vi "Test Tool Module API.vi"() -> ()   [LabVIEW 2015]
doc: "Tool Module API Tester.\n\n<b>Note:</b> This VI was modified by the <b>Validate DQMH Module</b> tool to upgrade it to the DQMH 3.0 approach to error handling in the tester VI, which avoids the potential for an error that stops the loop preventing the Stop Module VI from executing.\n\n<b>Note:</b> This VI was modified by the <b>Validate DQMH Module</b> tool to upgrade it to the DQMH 5.0 approach to only call the Stop Module.vi at the end of the tester if the module wasn't originally running when the tester started."
uses:
  Support/_STATUS Typedef--cluster.ctl
  GOTO Argument--cluster.ctl
  Support/_GoTo Cmd Typedef--enum.ctl
  Get All Inspect Data (Reply Payload)--cluster.ctl
  Tool Typedefs/_Temperature Threshold Arrays--typedef.ctl
  Return FPGA Setup Data (Reply Payload)--cluster.ctl
  Tool Typedefs/_FPGA Setup Params Cluster--typedef.ctl
  Tool Typedefs/_FPGA Timing Constraints Cluster--typedef.ctl
  Tool Typedefs/_FPGA Timing Ctrl Cluster--typedef.ctl
  Tool Typedefs/_FPGA Laser Config Cluster--typedef.ctl
  Tool Typedefs/_FPGA Peak Proc Cfg Cluster--typedef.ctl
  Tool Typedefs/_FPGA SPI Cfg Cluster--typedef.ctl
  Read from File Rtn Argument--cluster.ctl
  Tool Module.lvlib
  QC-X App/File Manager/File Manager.lvlib
panel:
  in  "Read Tool File":bool
  in  "Count":i32
  in  "Period":i32
  in  "Timer On":bool
  in  "Setup Timer 1":bool
  out "Return FPGA Setup Data":T1={"Version String"="", "FPGA Setup Parameters"={"FPGA Timing Constraints"={"frame.length Min"=530, "frame.ST_OFF Min"=15, "frame.ST_ON Min"=8, "frame.first data idx"=14, "frame.integ Offset"=6, "frame.integ Delay"=3, "frame.ad_latch Delay"=11, "frame.trig time Max"=0}, "FPGA Timing Ctrl"={"trig.time"=220, "integ.count 1"=400, "integ.count 2"=350, "encdr.latch ctrl"=1, "pixel.read count"=512, "clock.select"=2, "ad.clock offset"=16, "data.control reg"=2}, "FPGA Laser Config"={"laser.gain"=10, "laser.threshold Low"=1400, "laser.threshold High"=1900, "laser.dac init"=912, "laser.dac Min"=800, "laser.dac Max"=4000, "laser.config reg"=3}, "FPGA Peak Proc Cfg"={"PD.threshold"=0, "PD.width detect Min"=0, "PD.sensor pixels"=512, "PD.config reg"=23}, "FPGA SPI Cfg"={"SPI Divide Value"=1, "SPI config reg"=1}}, "Return FPGA Setup Data_error"={"status"=FALSE, "code"=0, "source"=""}} {"FPGA Setup Parameters"."FPGA SPI Cfg"."SPI config reg" format="%03b"; "FPGA Setup Parameters"."FPGA Peak Proc Cfg"."PD.config reg" format="%05b"; "FPGA Setup Parameters"."FPGA Laser Config"."laser.config reg" format="%02b"; "FPGA Setup Parameters"."FPGA Timing Ctrl"."data.control reg" format="%03b"; "FPGA Setup Parameters"."FPGA Timing Constraints"."frame.trig time Max" format="%0.0f"}
  in  "Return FPGA Setup Data":bool
  in  "Get Cycle Count":bool
  in  "Set Device Temp Tholds":bool
  in  "Device Temp Thold Arrays":T8
  in  "Read from File":bool
  in  "Write to File":bool
  out "error in (no error)":errorcluster
  out "XML String":string[](array[string])
  out "Waveform Graph":u16[][](graph)
  out "All Stop":bool
  out "Scan Data Array":u32[](array[numeric])
  out "Inspecting":bool
  out "Status 2":u8 format="%x"
  out "Reply Payload":T9
  out "Tool SN":u16
  out "Tool Type":u16
  out "Connected":bool
  in  "Get All Inspection Data":bool
  in  "Inspect Start/Stop":bool
  in  "Connect(T)/DisCon(F)":bool
  in  "INSPECT":bool
  in  "GOTO Button":bool caption="GOTO"
  in  "GOTO Cmd Params":T10
  out "Trigger":bool
  out "STATUS":T12
  in  "Tool Connect":bool
  in  "Show Block Diagram":bool
  in  "Stop Module":bool
  in  "Start Module":bool
  in  "Hide Module Panel":bool
  in  "Show Module Panel":bool
  out "Status":string
  out "Module Running?":bool
  # "This VI tests the API for the Module."
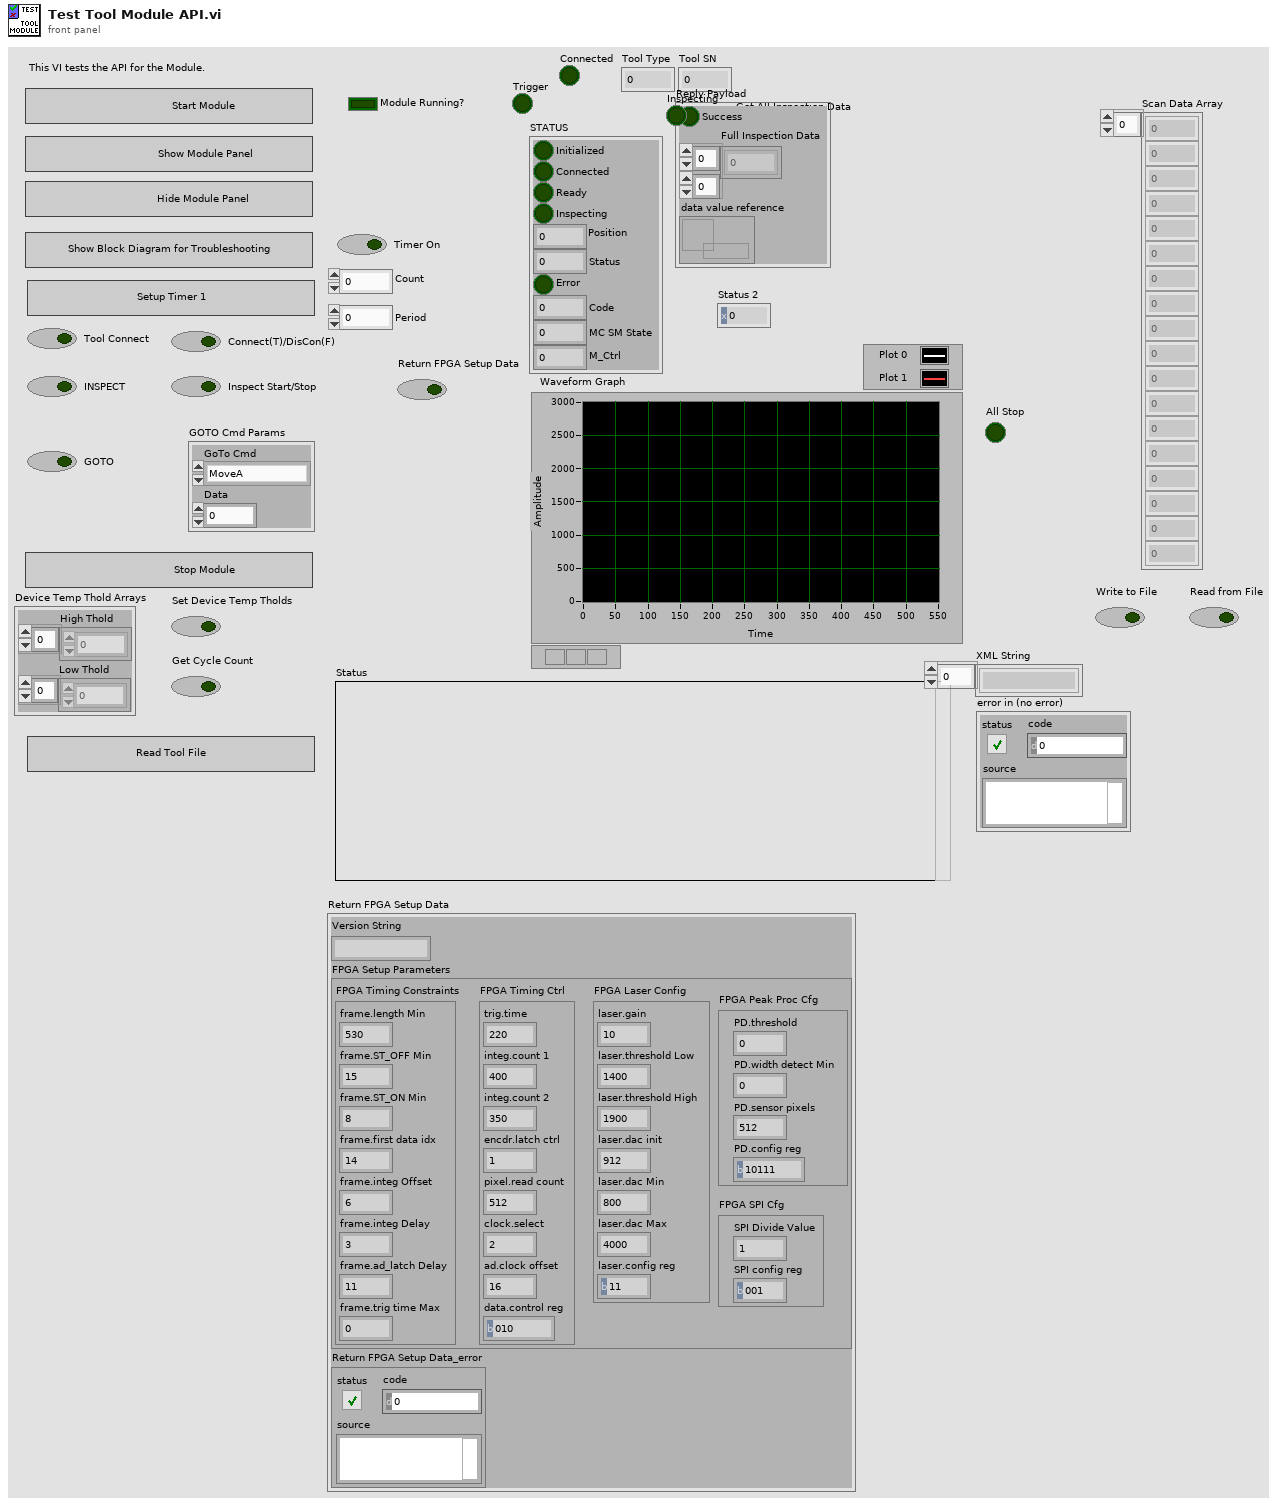
[diagram p1: front panel]
types:
  T1 = typedef "Tool Module.lvlib/Return FPGA Setup Data (Reply Payload)--cluster.ctl" = cluster{"Version String":string, "FPGA Setup Parameters":T2, "Return FPGA Setup Data_error":errorcluster}
  T2 = typedef "_FPGA Setup Params Cluster--typedef.ctl" = cluster{"FPGA Timing Constraints":T3, "FPGA Timing Ctrl":T4, "FPGA Laser Config":T5, "FPGA Peak Proc Cfg":T6, "FPGA SPI Cfg":T7}
  T3 = typedef "_FPGA Timing Constraints Cluster--typedef.ctl" = cluster{"frame.length Min":u16, "frame.ST_OFF Min":u16, "frame.ST_ON Min":u16, "frame.first data idx":u16, "frame.integ Offset":u16, "frame.integ Delay":u16, "frame.ad_latch Delay":u16, "frame.trig time Max":u32}
  T4 = typedef "_FPGA Timing Ctrl Cluster--typedef.ctl" = cluster{"trig.time":u32, "integ.count 1":u32, "integ.count 2":u32, "encdr.latch ctrl":u32, "pixel.read count":u16, "clock.select":u16, "ad.clock offset":u16, "data.control reg":u16}
  T5 = typedef "_FPGA Laser Config Cluster--typedef.ctl" = cluster{"laser.gain":i16, "laser.threshold Low":u16, "laser.threshold High":u16, "laser.dac init":u16, "laser.dac Min":u16, "laser.dac Max":u16, "laser.config reg":u16}
  T6 = typedef "_FPGA Peak Proc Cfg Cluster--typedef.ctl" = cluster{"PD.threshold":u16, "PD.width detect Min":u8, "PD.sensor pixels":u16, "PD.config reg":u16}
  T7 = typedef "_FPGA SPI Cfg Cluster--typedef.ctl" = cluster{"SPI Divide Value":u8, "SPI config reg":u16}
  T8 = typedef "_Temperature Threshold Arrays--typedef.ctl" = cluster{"High Thold ":dbl[], "Low Thold ":dbl[]}
  T9 = typedef "Tool Module.lvlib/Get All Inspect Data (Reply Payload)--cluster.ctl" = cluster{"Success":bool, "Full Inspection Data":u32[][], "data value reference":refnum<data-value>}
  T10 = typedef "Tool Module.lvlib/GOTO Argument--cluster.ctl" = cluster{"GoTo Cmd":T11, "Data":i32}
  T11 = typedef "Tool Module.lvlib/_GoTo Cmd Typedef--enum.ctl" = enum16{"MoveA", "MoveR", "Home Position", "Home None", "Cleaning Position"}
  T12 = typedef "Tool Module.lvlib/_STATUS Typedef--cluster.ctl" = cluster{"Initialized":bool, "Connected":bool, "Ready":bool, "Inspecting":bool, "Position":dbl, "Status":u16, "Error":bool, "Code":i32, "MC SM State":u16, "M_Ctrl":u16}
  T13 = typedef "Tool Module.lvlib/Broadcast Events--cluster.ctl" = cluster{"Module Did Init":refnum<user-event>, "Status Updated":refnum<user-event>, "Error Reported":refnum<user-event>, "Module Did Stop":refnum<user-event>, "Update Module Execution Status":refnum<user-event>, "Send Status":refnum<user-event>, "Trigger":refnum<user-event>, "Connected":refnum<user-event>, "Read from File Rtn":refnum<user-event>, "Device Temperature":refnum<user-event>, "Time Expired":refnum<user-event>}
  T14 = typedef "Tool Module.lvlib/_Sample Data Rtn Cluster--typedef.ctl" = cluster{"InspectCycle":bool, "Acquiring Data":bool, "Sample Available":bool, "Scan Complete":bool, "Cancelled":bool, "Scan Data Array":u32[], "error cluster":errorcluster}
  T15 = typedef "Tool Module.lvlib/Read from File Rtn Argument--cluster.ctl" = cluster{"Filename":string, "XML Strings":string[], "Error Status":errorcluster}
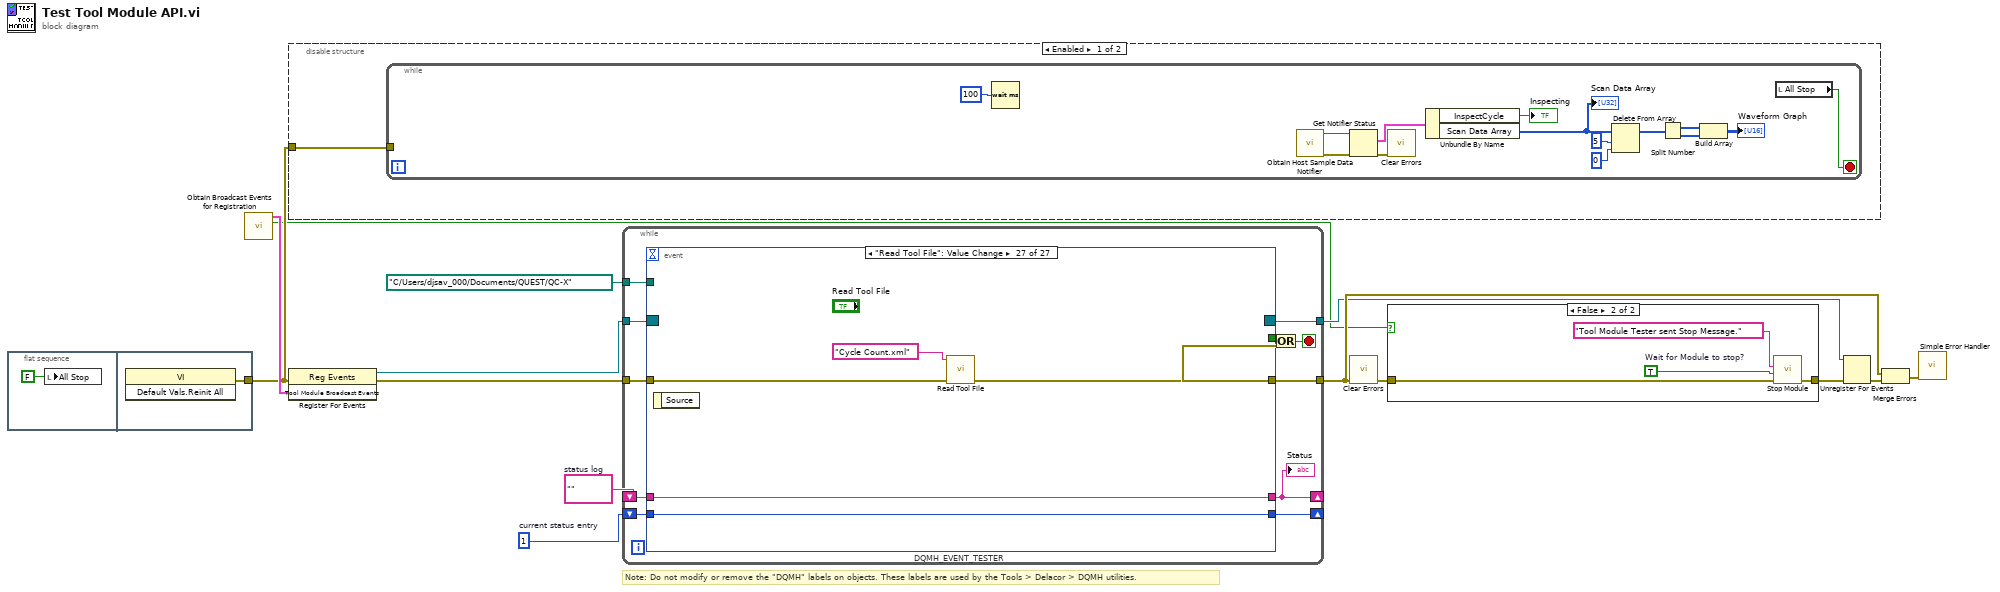
[diagram p0: block diagram]
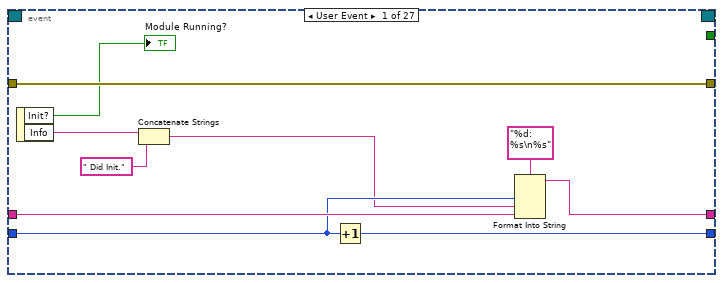
[diagram p4: hidden frame]
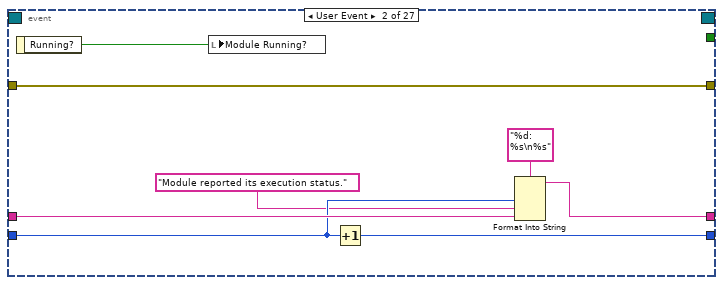
[diagram p5: hidden frame]
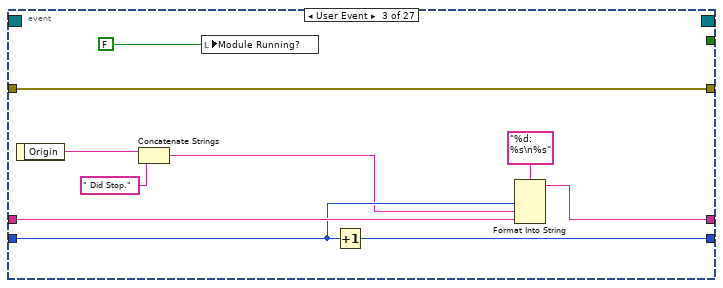
[diagram p6: hidden frame]
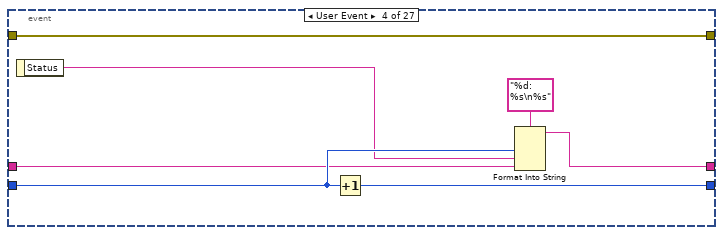
[diagram p7: hidden frame]
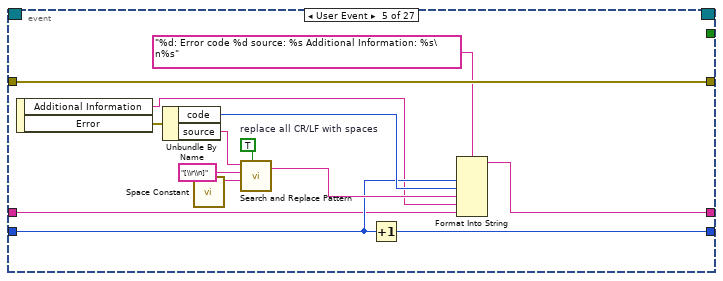
[diagram p8: hidden frame]
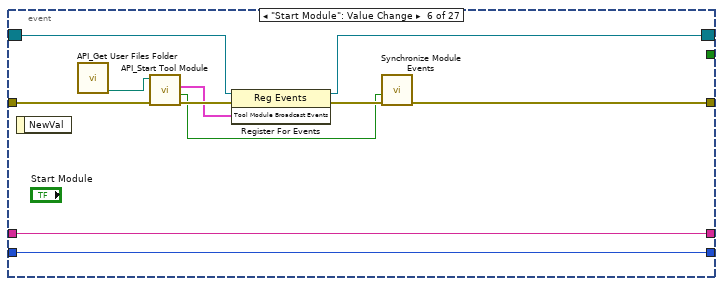
[diagram p9: hidden frame]
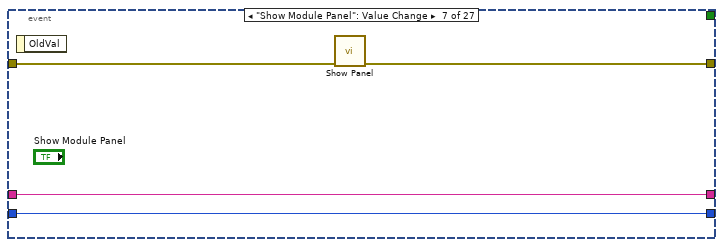
[diagram p10: hidden frame]
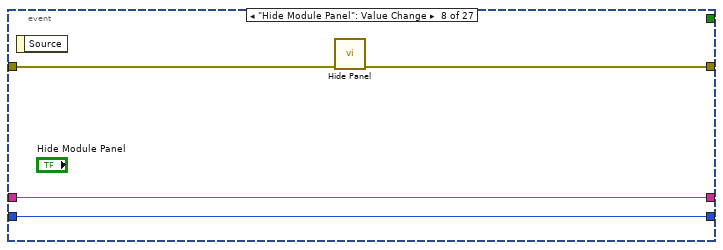
[diagram p11: hidden frame]
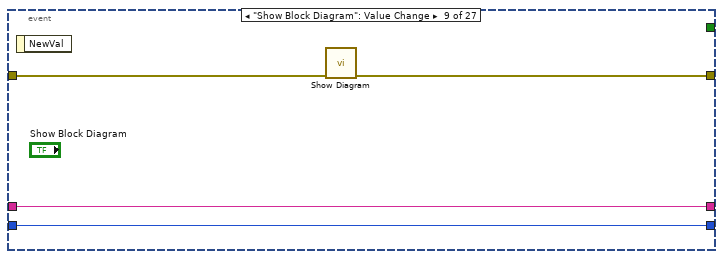
[diagram p12: hidden frame]
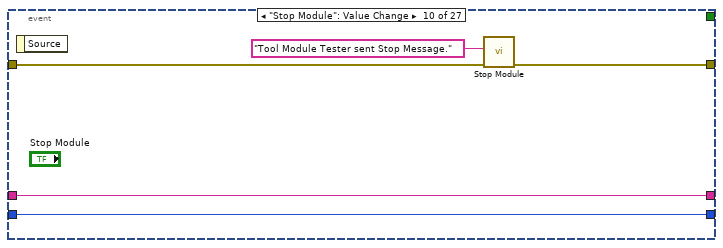
[diagram p13: hidden frame]
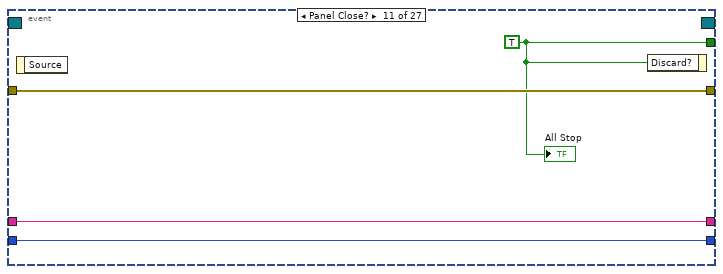
[diagram p14: hidden frame]
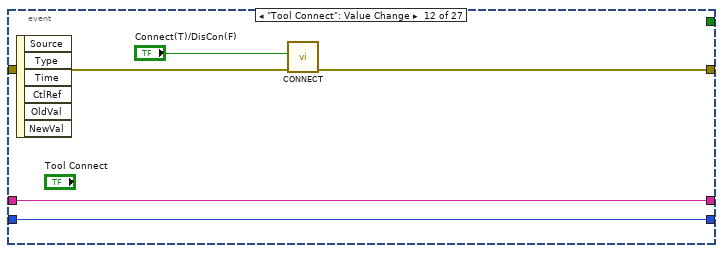
[diagram p15: hidden frame]
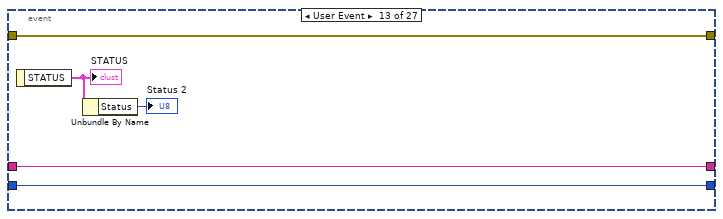
[diagram p16: hidden frame]
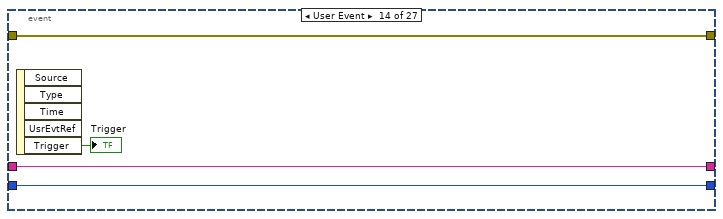
[diagram p17: hidden frame]
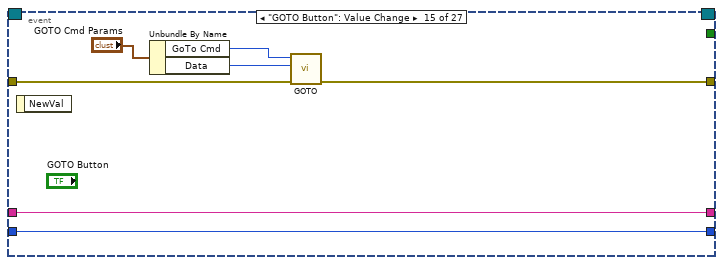
[diagram p18: hidden frame]
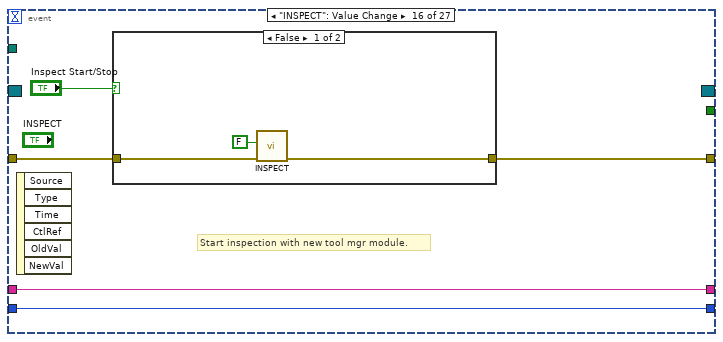
[diagram p19: hidden frame]
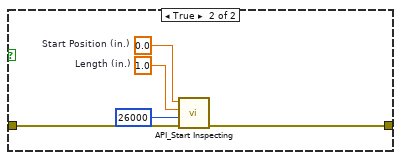
[diagram p20: hidden frame]
diagram:
  w10 = 1  # current status entry
  w11 = ""  # status log
  # "Note: Do not modify or remove the \"DQMH\" labels on objects. These labels are used by the Tools > Delacor > DQMH utilities."
  n1 = flat-sequence {
    tunnel: [w16] -> w4
    frame #0 {
      n2 = local write "All Stop"(FALSE ("All Stop")) -> ()
    }
    frame #1 {
      n3 = invoke class="VI" method="Default Vals.Reinit All"() -> (error out=w16:errorcluster)  [unwired: 3 in, 2 out]
    }
  }
  n4 = call "Obtain Broadcast Events for Registration.vi"() -> ("Already running?"=w1:bool, "Tool Module Broadcast Events"=w8:T13)  [unwired: 9 in, 1 out]
  n5 = disable-structure shown="Enabled" {
    disable-tunnel: w4 -> [w17 _]
    frame Enabled {
      n6 = while {
        tunnel: w17 -> [_]
        stop <- w26 stop-if-true
        n7 = Wait (ms)(milliseconds to wait=u32 100) -> ()  [unwired: 1 out]
        n8 = call "Obtain Host Sample Data Notifier.vi"() -> ("error out"=w29:errorcluster, "Sample Data Notifier"=w18:refnum<notifier>)  [unwired: 10 in]
        n9 = Get Notifier Status(notifier=w18, error in (no error)=w29) -> (current notification=w28:T14, error out=w31:errorcluster)  [unwired: 3 out]
        n10 = call <vilib>:"Clear Errors.vi"("error in (no error)"=w31) -> ()  [unwired: 5 in, 2 out]
        n11 = Unbundle By Name(w28) -> ("InspectCycle"=→"Inspecting":bool, "Scan Data Array"=w25:u32[])
        "Scan Data Array" <- w25
        n12 = Delete From Array(array=w25, length=5, index=0) -> (array with subset deleted=w22:u32[])  [unwired: 1 out]
        n13 = Split Number(x=w22) -> (hi(x)=w21:u16[], lo(x)=w20:u16[])
        n14 = Build Array(w21, w20) -> (→"Waveform Graph":u16[][])
        n15 = local read "All Stop"() -> (w26:bool)
      }
    }
    frame Disabled {
    }
  }
  n16 = register-events(error in=w4, w8) -> (reference out=w7:refnum<event-registration>, error out=w9:errorcluster)  [unwired: 1 in]
  n17 = while {
    tunnel: w7 -> [w42]
    tunnel: [w35] -> w12
    shift-right: [w37] -> _
    shift-left: w11 -> [w39]
    shift-right: [w38] -> _
    shift-left: w10 -> [w40]
    tunnel: w9 -> [w34]
    tunnel: [w33] -> w6
    tunnel: path "C:/Users/djsav_000/Documents/QUEST/QC-X" ("Cfg File Path") -> [w32]
    stop <- w36 stop-if-true
    n18 = event "DQMH_EVENT_TESTER" shown="[26] \"Read Tool File\": Value Change" {
      selector: w42 -> [_ _ _ _ _ w96 _ _ _ _ _ _ _ _ _ _ _ _ _ _ _ _ _ _ _ _ _]
      dyn-events: [_ _ _ _ _ w95 _ _ _ _ _ _ _ _ _ _ _ _ _ _ _ _ _ _ _ _ _] -> w33
      timeout: _ -> [_ _ _ _ _ _ _ _ _ _ _ _ _ _ _ _ _ _ _ _ _ _ _ _ _ _ _]
      tunnel: [_ _ _ _ _ _ _ _ _ _ w120 _ _ _ _ _ _ _ _ _ _ _ _ _ _ _ _] -> w41
      tunnel: [w52 w54 w61 w71 w91 w94 w106 w110 w111 w117 w121 w124 w133 w137 w141 w146 w169 w175 w183 w187 w192 w198 w200 w205 w210 w217 w228] -> w35
      tunnel: w40 -> [w48 w58 w68 w74 w81 w99 w104 w108 w112 w118 w122 w127 w131 w135 w142 w148 w166 w176 w181 w188 w193 w196 w201 w206 w211 w218 w229]
      tunnel: w39 -> [w49 w59 w69 w73 w79 w100 w105 w109 w113 w119 w123 w128 w132 w136 w143 w149 w165 w177 w182 w189 w194 w197 w202 w207 w212 w219 w230]
      tunnel: [w46 w56 w66 w75 w82 w100 w105 w109 w113 w119 w123 w128 w132 w136 w143 w149 w161 w177 w182 w189 w194 w197 w202 w207 w212 w219 w230] -> w37
      tunnel: [w47 w57 w67 w77 w80 w99 w104 w108 w112 w118 w122 w127 w131 w135 w142 w148 w167 w176 w181 w188 w193 w196 w201 w206 w211 w218 w229] -> w38
      tunnel: w34 -> [w52 w54 w61 w71 w91 w93 w103 w107 w114 w115 w121 w126 w133 w137 w144 w147 w169 w178 w183 w190 w195 w198 w203 w208 w213 w220 w231]
      tunnel: w32 -> [_ _ _ _ _ _ _ _ _ _ _ _ _ _ _ _ _ _ _ _ _ _ _ _ _ _ _]
      event User Event {
        n19 = event-data() -> ("Init?"=→"Module Running?":bool, "Info"=w45:string)  [unwired: 1 in]
        n20 = Concatenate Strings(w45, " Did Init.") -> (w44:string)
        n21 = Increment(x=w48) -> (x+1=w47:i32)
        n22 = Format Into String(format string="%d: %s\n%s", w48, w44, w49) -> (resulting string=w46:string)  [unwired: 2 in, 1 out]
      }
      event User Event {
        n23 = event-data() -> ("Running?"=w53:bool)  [unwired: 1 in]
        n24 = local write "Module Running?"(w53) -> ()
        n25 = Increment(x=w58) -> (x+1=w57:i32)
        n26 = Format Into String(format string="%d: %s\n%s", w58, "Module reported its execution status.", w59) -> (resulting string=w56:string)  [unwired: 2 in, 1 out]
      }
      event User Event {
        n27 = event-data() -> ("Origin"=w65:string)  [unwired: 1 in]
        n28 = Concatenate Strings(w65, " Did Stop.") -> (w64:string)
        n29 = local write "Module Running?"(FALSE ("Module Did Init?")) -> ()
        n30 = Increment(x=w68) -> (x+1=w67:i32)
        n31 = Format Into String(format string="%d: %s\n%s", w68, w64, w69) -> (resulting string=w66:string)  [unwired: 2 in, 1 out]
      }
      event User Event {
        n32 = event-data() -> ("Status"=w72:string)  [unwired: 1 in]
        n33 = Increment(x=w74) -> (x+1=w77:i32)
        n34 = Format Into String(format string="%d: %s\n%s", w74, w72, w73) -> (resulting string=w75:string)  [unwired: 2 in, 1 out]
      }
      event User Event {
        w87 = TRUE  # replace all CR/LF with spaces
        n35 = event-data() -> ("Additional Information"=w78:string, "Error"=w83:errorcluster)  [unwired: 1 in]
        n36 = Unbundle By Name(w83) -> ("code"=w84:i32, "source"=w85:string)
        n37 = call <vilib>:"Space Constant.vi"() -> ("String"=w88:string)
        n38 = call <vilib>:"Search and Replace Pattern.vi"("string"=w85, "regular expression (\"\")"="[\\r\\n]" ("regular expression (\"\")"), "replace string (\"\")"=w88, "replace all? (F)"=w87) -> ("result string"=w86:string)  [unwired: 1 in, 1 out]
        n39 = Increment(x=w81) -> (x+1=w80:i32)
        n40 = Format Into String(format string="%d: Error code %d source: %s Additional Information: %s\n%s", w81, w84, w86, w78, w79) -> (resulting string=w82:string)  [unwired: 2 in, 1 out]
      }
      event "Start Module": Value Change {
        n41 = event-data() -> ()  [unwired: 1 in, 1 out]
        n42 = call "API_Get User Files Folder.vi"() -> ("App Setup Filename"=w92:path)  [unwired: 5 in, 6 out]
        n43 = call "API_Start Tool Module.vi"("error in (no error)"=w93, "Cfg File Path"=w92) -> ("error out"=w101:errorcluster, "Wait for Event Sync?"=w98:bool, "Tool Module Broadcast Events"=w97:T13)  [unwired: 7 in]
        n44 = register-events(reference=w96, error in=w101, w97) -> (reference out=w95:refnum<event-registration>, error out=w102:errorcluster)
        n45 = call "Synchronize Module Events.vi"("error in (no error)"=w102, "Wait for Event Sync?"=w98) -> ("error out"=w94:errorcluster)  [unwired: 9 in]
      }
      event "Show Module Panel": Value Change {
        n46 = event-data() -> ()  [unwired: 1 in, 1 out]
        n47 = call "Show Panel.vi"("error in (no error)"=w103) -> ("error out"=w106:errorcluster)  [unwired: 10 in]
      }
      event "Hide Module Panel": Value Change {
        n48 = event-data() -> ()  [unwired: 1 in, 1 out]
        n49 = call "Hide Panel.vi"("error in (no error)"=w107) -> ("error out"=w110:errorcluster)  [unwired: 10 in]
      }
      event "Show Block Diagram": Value Change {
        n50 = event-data() -> ()  [unwired: 1 in, 1 out]
        n51 = call "Show Diagram.vi"("error in (no error)"=w114) -> ("error out"=w111:errorcluster)  [unwired: 10 in]
      }
      event "Stop Module": Value Change {
        n52 = event-data() -> ()  [unwired: 1 in, 1 out]
        n53 = call "Stop Module.vi"("error in (no error)"=w115, "Origin"="Tool Module Tester sent Stop Message.") -> ("error out"=w117:errorcluster)  [unwired: 9 in]
      }
      event Panel Close? {
        w120 = TRUE ("Discard?")
        n54 = event-data() -> ()  [unwired: 1 in, 1 out]
        n55 = event-data("Discard?"=w120) -> ()  [unwired: 1 in, 1 out]
        "All Stop" <- w120
      }
      event "Tool Connect": Value Change {
        n56 = event-data() -> ()  [unwired: 1 in, 6 out]
        n57 = call "CONNECT.vi"("error in (no error)"=w126, "Connect"="Connect(T)/DisCon(F)") -> ("error out"=w124:errorcluster)  [unwired: 9 in]
      }
      event User Event {
        n58 = event-data() -> ("STATUS"=w130:T12)  [unwired: 1 in]
        "STATUS" <- w130
        n59 = Unbundle By Name(w130) -> ("Status"=→"Status 2":u16)
      }
      event User Event {
        n60 = event-data() -> ("Trigger"=→"Trigger":bool)  [unwired: 1 in, 4 out]
      }
      event "GOTO Button": Value Change {
        n61 = event-data() -> ()  [unwired: 1 in, 1 out]
        n62 = Unbundle By Name("GOTO Cmd Params") -> ("GoTo Cmd"=w139:T11, "Data"=w138:i32)
        n63 = call "GOTO.vi"("error in (no error)"=w144, "Data"=w138, "GoTo Cmd"=w139) -> ("error out"=w141:errorcluster)  [unwired: 8 in]
      }
      event "INSPECT": Value Change {
        # "Start inspection with new tool mgr module."
        n64 = event-data() -> ()  [unwired: 1 in, 6 out]
        n65 = case shown="False" "Inspect Start/Stop" {
          tunnel: w147 -> [w152 w157]
          tunnel: [w151 w153] -> w146
          frame False {
            n66 = call "INSPECT.vi"("error in (no error)"=w152, "Start(T)/Stop(F)"=FALSE) -> ("error out"=w151:errorcluster)  [unwired: 7 in, 2 out]
          }
          frame True {
            w155 = 1.0  # Length (in.)
            w156 = 0.0  # Start Position (in.)
            n67 = call "API_Start Inspecting.vi"("error in (no error)"=w157, "Samples Per Inch"=26000 ("Max Samples"), "Inspect.Length (in.)"=w155, "Inspect.Start (in.)"=w156) -> ("error out"=w153:errorcluster)  [unwired: 3 in, 4 out]
          }
        }
      }
      event User Event {
        n68 = event-data() -> ("Connected"=w158:bool, "Tool Type"=→"Tool Type":u16, "Tool SN"=→"Tool SN":u16)  [unwired: 1 in, 4 out]
        "Connected" <- w158
        n69 = case shown="False" w158 {
          frame False {
            w171 = FALSE ("Initialized")
            n70 = local read "STATUS"() -> (w172:T12)
            n71 = Bundle By Name(cluster=w172, "Initialized"=w171, "Connected"=w171, "Ready"=w171, "Inspecting"=w171) -> (w170:T12)
            n72 = local write "STATUS"(w170) -> ()
          }
          frame True {
          }
        }
        n73 = Select(t="Tool Connected", s=w158, f="Tool Disconnected") -> (s? t:f=w162:string)
        n74 = Increment(x=w166) -> (x+1=w167:i32)
        n75 = Format Into String(format string="%d: %s\n%s", w166, w162, w165) -> (resulting string=w161:string)  [unwired: 2 in, 1 out]
      }
      event "Get All Inspection Data": Value Change {
        n76 = event-data() -> ()  [unwired: 1 in, 6 out]
        n77 = call "Get All Inspect Data.vi"("error in (no error)"=w178, "dummy"="Get All Inspection Data") -> ("error out"=w175:errorcluster, "Reply Payload"=→"Reply Payload":T9)  [unwired: 7 in, 1 out]
      }
      event User Event {
        n78 = event-data() -> ("XML Strings"=→"XML String":string[], "Error Status"=→"error in (no error)":errorcluster)  [unwired: 1 in, 4 out]
      }
      event "Write to File": Value Change {
        (unwired) cluster{"No.":i32, "YMax":dbl} {"No."=0, "YMax"=0.0}
        n79 = event-data() -> ()  [unwired: 1 in, 6 out]
        n80 = Flatten To XML(anything=T15 {"Filename"="", "XML Strings"=[], "Error Status"={"status"=FALSE, "code"=0, "source"=""}} ("Read from File Rtn Argument")) -> ()  [unwired: 1 out]
        n81 = call "Write to File.vi"("error in (no error)"=w190, "Flattened data strings"=string[] [], "Filename"="Test.xml") -> ("error out"=w187:errorcluster)  [unwired: 8 in]
      }
      event "Read from File": Value Change {
        n82 = event-data() -> ()  [unwired: 1 in, 6 out]
        n83 = call "Read from File.vi"("error in (no error)"=w195, "Filename"="Cycle Count.xml") -> ("error out"=w192:errorcluster)  [unwired: 9 in]
      }
      event User Event {
        n84 = event-data() -> ()  [unwired: 1 in, 5 out]
      }
      event "Set Device Temp Tholds": Value Change {
        n85 = event-data() -> ()  [unwired: 1 in, 6 out]
        n86 = call "Set Device Temp Thresholds.vi"("error in (no error)"=w203, "Device Temp Thold Arrays"="Device Temp Thold Arrays") -> ("error out"=w200:errorcluster)  [unwired: 9 in]
      }
      event "Get Cycle Count": Value Change {
        w204 = FALSE  # Clear?
        n87 = event-data() -> ()  [unwired: 1 in, 6 out]
        n88 = call "Get Cycle Count.vi"("error in (no error)"=w208, "Clear?"=w204) -> ("error out"=w205:errorcluster)  [unwired: 7 in, 2 out]
      }
      event "Return FPGA Setup Data": Value Change {
        n89 = event-data() -> ()  [unwired: 1 in, 6 out]
        n90 = call "Return FPGA Setup Data.vi"("error in (no error)"=w213) -> ("error out"=w210:errorcluster, "Reply Payload"=→"Return FPGA Setup Data":T1)  [unwired: 8 in, 1 out]
      }
      event "Setup Timer 1": Value Change {
        # "Make request vi public to use."
        n91 = event-data() -> ()  [unwired: 1 in, 1 out]
        n92 = disable-structure shown="Disabled" {
          disable-tunnel: w220 -> [w225 w226]
          disable-tunnel: [w224 w226] -> w217
          disable-tunnel: "Timer On" -> [w223 _]
          disable-tunnel: "Period" -> [w222 _]
          disable-tunnel: "Count" -> [w221 _]
          frame Disabled {
            n93 = call "Setup Timer.vi"("error in (no error)"=w225, "Count"=w221, "Period"=w222, "Timer On"=w223) -> ("error out"=w224:errorcluster)  [unwired: 7 in]
          }
          frame Enabled {
          }
        }
      }
      event "Read Tool File": Value Change {
        n94 = event-data() -> ()  [unwired: 1 in, 1 out]
        n95 = call "Read Tool File.vi"("error in (no error)"=w231, "Filename"="Cycle Count.xml") -> ("error out"=w228:errorcluster)  [unwired: 7 in, 2 out]
      }
    }
    "Status" <- w37
    n96 = Or(x=w41, y=w35) -> (x .or. y?=w36:bool)
  }
  n97 = call <vilib>:"Clear Errors.vi"("error in (no error)"=w12) -> ("error out"=w3:errorcluster)  [unwired: 5 in, 1 out]
  n98 = case shown="False" w1 {
    tunnel: [w232 w236] -> w13
    tunnel: w3 -> [w232 w233]
    frame True {
    }
    frame False {
      w234 = TRUE  # Wait for Module to stop?
      n99 = call "Stop Module.vi"("error in (no error)"=w233, "Wait for Module to Stop? (F)"=w234, "Origin"="Tool Module Tester sent Stop Message.") -> ("error out"=w236:errorcluster)  [unwired: 8 in]
    }
  }
  n100 = Unregister For Events(event registration refnum=w6, error in=w13) -> (error out=w14:errorcluster)
  n101 = Merge Errors(w12, w14) -> (w2:errorcluster)
  n102 = call <vilib>:"Simple Error Handler.vi"("error in (no error)"=w2) -> ()  [unwired: 4 in, 5 out]
